vi "Listbox data filter.vi"(11 "ProgramData":T1={"Tytuły"=[], "Folder"=path "", "Data/tytul"=[], "Ostatni index"=-10, "Title"="", "Note"=""}) -> (3 "Array":string[](array[string]))   [LabVIEW 2020]
uses:
  #typeDef_ProgramData.ctl
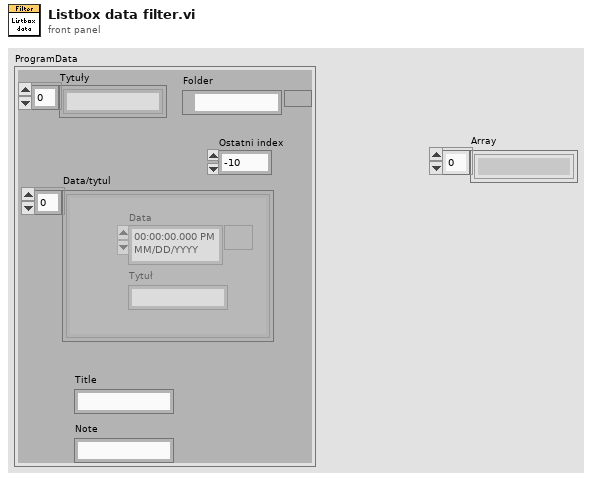
[diagram p1: front panel]
types:
  T1 = typedef "#typeDef_ProgramData.ctl" = cluster{"Tytuły":string[], "Folder":path, "Data/tytul":cluster{"Data":timestamp, "Tytuł":string}[], "Ostatni index":i32, "Title":string, "Note":string}
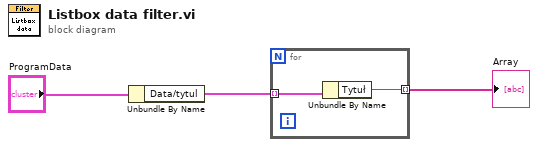
[diagram p0: block diagram]
diagram:
  n1 = Unbundle By Name("ProgramData") -> ("Data/tytul"=w2:cluster{"Data":timestamp, "Tytuł":string}[])
  n2 = for {
    tunnel: w2 -> [w5] mode=indexing
    tunnel: [w4] -> w1 mode=indexing
    n3 = Unbundle By Name(w5) -> ("Tytuł"=w4:string)
  }
  "Array" <- w1
